vi "Periodic Tasks.vi"(8 "error in":errorcluster) -> ()   [LabVIEW 2019]
doc: "This VI runs in parallel to other tasks. It can contain as many user-defined periodic loops as you need. These can carry out PID or other sorts of timed response."
uses:
  <vilib>/Rock Robotics/WPI/DriverStation/WPI_DriverStationRobotMode2.ctl
  <vilib>/Rock Robotics/WPI/Utilities/WPI_GetSetVariantRefNum.vi
  Robot Global Data.vi
  <vilib>/Rock Robotics/WPI/RobotDrive/WPI_RobotDriveArcadeDrive_Standard(NoSaturation).vi
  <vilib>/Rock Robotics/Network Tables/NT Write Numeric Array.vi
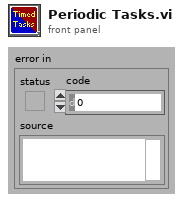
[diagram p1: front panel]
types:
  T1 = typedef "WPI_RobotDriveDevRef.ctl" = cluster{"DevStatus":errorcluster, "Motors[]":T2[], "Square Inputs":bool, "Max Output":dbl}
  T2 = typedef "WPI_MotorControlDeviceRef.ctl" = cluster{"DeviceStatus":errorcluster, "Type":T3, "PWM":cluster{"PWM Channel":T4, "DeadBand":T5}, "CAN":cluster{"Device Number":u8, "SetOutput VI Ref":variant, "GetOutput VI Ref":variant, "Enable VI Ref":variant, "Disable VI Ref":variant, "Data":variant}, "Invert":bool, "DIO PWM":cluster{"PWM \"Enable\" Channel":T4, "DIOChannel":T6, "PWM Rate":dbl}}
  T3 = typedef "WPI_MotorControlType.ctl" = enum16{"PWM", "CAN", "DIO PWM"}
  T4 = typedef "FPGA_DIOPWMChannel.ctl" = enum8{"PWM 0", "PWM 1", "PWM 2", "PWM 3", "PWM 4", "PWM 5", "PWM 6", "PWM 7", "PWM 8", "PWM 9", "PWM MXP 0", "PWM MXP 1", "PWM MXP 2", "PWM MXP 3", "PWM MXP 4", "PWM MXP 5", "PWM MXP 6", "PWM MXP 7", "PWM MXP 8", "PWM MXP 9", "Invalid"}
  T5 = typedef "WPI_PWMDeadband.ctl" = cluster{"Name":string, "maxPositivePwm":i32, "minPositivePwm":i32, "centerPwm":i32, "maxNegativePwm":i32, "minNegativePwm":i32, "angularRange":u16}
  T6 = typedef "FPGA_DIOChannel.ctl" = enum8{"DIO 0", "DIO 1", "DIO 2", "DIO 3", "DIO 4", "DIO 5", "DIO 6", "DIO 7", "DIO 8", "DIO 9", "DIO MXP 0", "DIO MXP 1", "DIO MXP 2", "DIO MXP 3", "DIO MXP 4", "DIO MXP 5", "DIO MXP 6", "DIO MXP 7", "DIO MXP 8", "DIO MXP 9", "DIO MXP 10", "DIO MXP 11", "DIO MXP 12", "DIO MXP 13", "DIO MXP 14", "DIO MXP 15", "SPI Port CS1", "SPI Port CS2", "SPI Port CS3", "SPI Port MISO", "SPI Port MOSI", "Invalid"}
  T7 = typedef "WPI_JoystickDevRef.ctl" = cluster{"Device":T8}
  T8 = typedef "WPI_JoystickDeviceEnum.ctl" = enum16{"USB 0", "USB 1", "USB 2", "USB 3", "USB 4", "USB 5"}
  T9 = cluster{"JoystickDevRef":T7, "RobotDriveDevRef":T1}
  T10 = typedef "WPI_DriverStationRobotMode2.ctl" = enum16{"Autonomous Disabled", "Autonomous Enabled", "Teleop Disabled", "Teleop Enabled", "Disconnected", "Finish", "Test Disabled", "Test Enabled", "Emergency Stopped"}
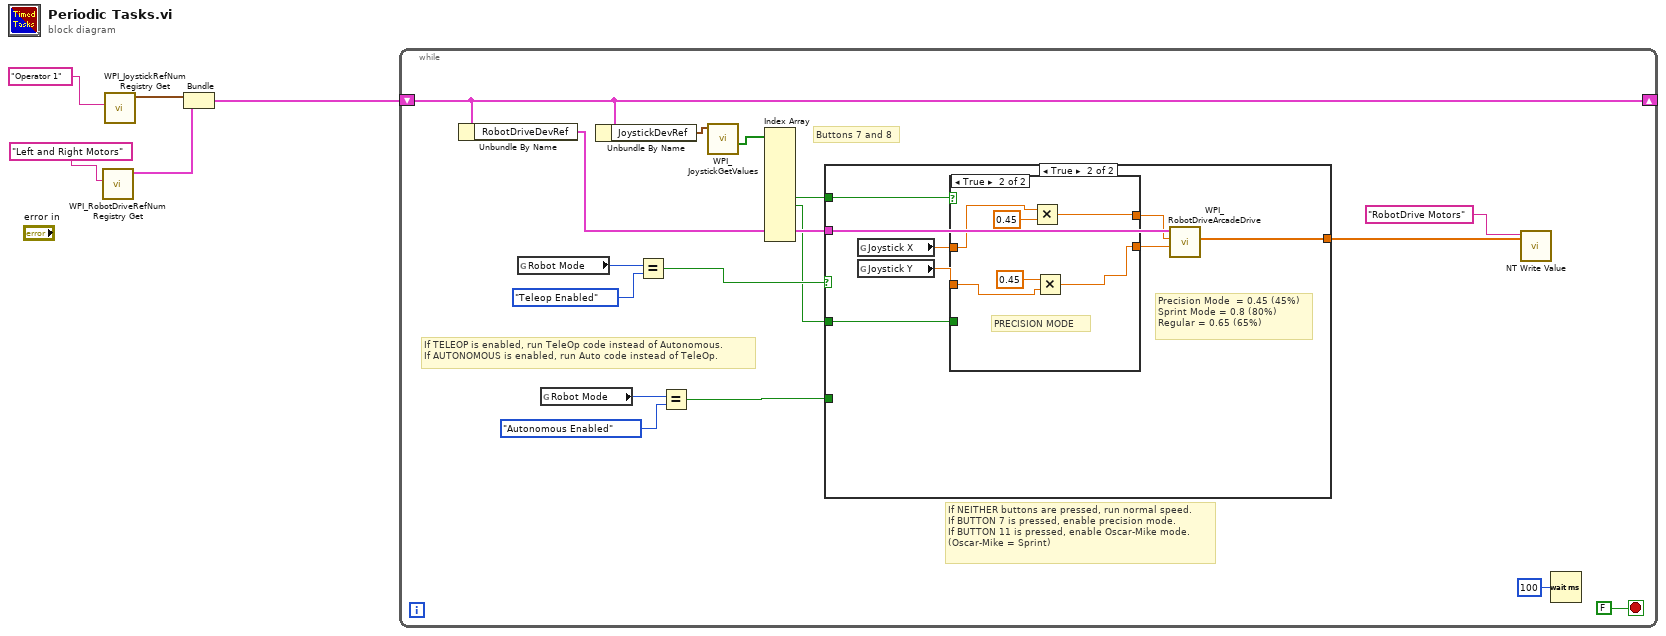
[diagram p0: block diagram]
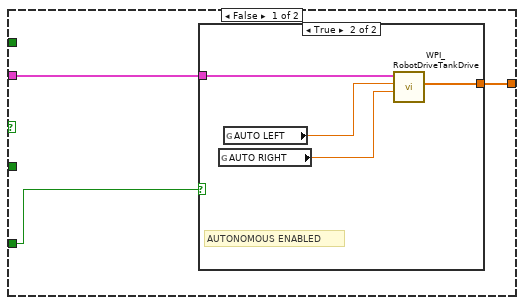
[diagram p2: hidden frame]
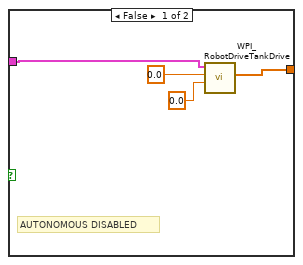
[diagram p3: hidden frame]
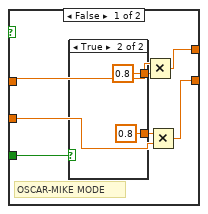
[diagram p4: hidden frame]
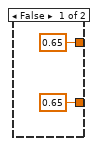
[diagram p5: hidden frame]
diagram:
  n1 = call <vilib>:"WPI_RobotDriveRefNum Registry Get.vi"("refnum name"="Left and Right Motors") -> ("RobotDriveDevRef"=w5:T1)  [unwired: 1 in, 9 out]
  n2 = call <vilib>:"WPI_JoystickRefNum Registry Get.vi"("refnum name"="Operator 1") -> ("JoystickDevRef"=w4:T7)  [unwired: 1 in, 9 out]
  n3 = Bundle("JoystickDevRef"=w4, "RobotDriveDevRef"=w5) -> (w1:T9)  [unwired: 1 out]
  n4 = while {
    shift-right: [w10] -> _
    shift-left: w1 -> [w10]
    stop <- FALSE stop-if-true
    # "If NEITHER buttons are pressed, run normal speed.\nIf BUTTON 7 is pressed, enable precision mode.\nIf BUTTON 11 is pressed, enable Oscar-Mike mode.\n(Oscar-Mike = Sprint)"
    # "Buttons 7 and 8"
    # "If TELEOP is enabled, run TeleOp code instead of Autonomous.\nIf AUTONOMOUS is enabled, run Auto code instead of TeleOp."
    n5 = Unbundle By Name(w10) -> ("RobotDriveDevRef"=w17:T1)
    n6 = global read "Robot Global Data.vi" "Robot Mode"() -> (w15:T10)
    n7 = global read "Robot Global Data.vi" "Robot Mode"() -> (w13:T10)
    n8 = Unbundle By Name(w10) -> ("JoystickDevRef"=w9:T7)
    n9 = Equal?(x=w15, y=WPI_DriverStationRobotMode2."Teleop Enabled") -> (x = y?=w16:bool)
    n10 = Equal?(x=w13, y=WPI_DriverStationRobotMode2."Autonomous Enabled") -> (x = y?=w11:bool)
    n11 = call <vilib>:"WPI_JoystickGetValues.vi"("JoystickDevRef"=w9) -> ("Buttons"=w8:bool[])  [unwired: 6 in, 4 out]
    n12 = Index Array(array=w8) -> (element #7=w7:bool, element #8=w6:bool)  [unwired: 12 in, 10 out]
    n13 = case shown="True" w16 {
      tunnel: [w24 w39] -> w18
      tunnel: w17 -> [w23 w40]
      tunnel: w11 -> [w22 _]
      tunnel: w6 -> [_ w34]
      tunnel: w7 -> [_ w33]
      frame False {
        n14 = case shown="True" w22 {
          tunnel: [w28 w32] -> w24
          tunnel: w23 -> [w25 w30]
          frame False {
            # "AUTONOMOUS DISABLED"
            n15 = call <vilib>:"WPI_RobotDriveTankDrive.vi"("Right axis value"=0.0, "Left axis value"=0.0, "RobotDriveDevRef"=w25) -> ("Motor Values"=w28:dbl[])  [unwired: 6 in, 2 out]
          }
          frame True {
            # "AUTONOMOUS ENABLED"
            n16 = global read "Robot Global Data.vi" "AUTO RIGHT"() -> (w29:dbl)
            n17 = global read "Robot Global Data.vi" "AUTO LEFT"() -> (w31:dbl)
            n18 = call <vilib>:"WPI_RobotDriveTankDrive.vi"("Right axis value"=w29, "Left axis value"=w31, "RobotDriveDevRef"=w30) -> ("Motor Values"=w32:dbl[])  [unwired: 6 in, 2 out]
          }
        }
      }
      frame True {
        # "Precision Mode  = 0.45 (45%)\nSprint Mode = 0.8 (80%)\nRegular = 0.65 (65%)"
        n19 = global read "Robot Global Data.vi" "Joystick X"() -> (w38:dbl)
        n20 = global read "Robot Global Data.vi" "Joystick Y"() -> (w37:dbl)
        n21 = case shown="True" w33 {
          tunnel: w38 -> [w44 w55]
          tunnel: w37 -> [w45 w54]
          tunnel: [w43 w56] -> w36
          tunnel: [w42 w57] -> w35
          tunnel: w34 -> [w41 _]
          frame False {
            # "OSCAR-MIKE MODE"
            n22 = case shown="True" w41 {
              tunnel: [0.65 ("x") 0.8 ("x")] -> w47
              tunnel: [0.65 ("y") 0.8 ("y")] -> w46
              frame False {
              }
              frame True {
              }
            }
            n23 = Multiply(x=w44, y=w46) -> (x*y=w43:dbl)
            n24 = Multiply(x=w47, y=w45) -> (x*y=w42:dbl)
          }
          frame True {
            # "PRECISION MODE"
            n25 = Multiply(x=w55, y=0.45) -> (x*y=w56:dbl)
            n26 = Multiply(x=0.45, y=w54) -> (x*y=w57:dbl)
          }
        }
        n27 = call-poly <vilib>:"WPI_RobotDriveArcadeDrive.vi"("Y axis value"=w35, "X axis value"=w36, "RobotDriveDevRef"=w40) -> ("Motor Values"=w39:dbl[])  [unwired: 6 in, 2 out]
      }
    }
    n28 = call-poly <vilib>:"NT Write Value.vi"("Numeric Array"=w18, "Name"="RobotDrive Motors") -> ()  [unwired: 9 in, 1 out]
    n29 = Wait (ms)(milliseconds to wait=u32 100) -> ()  [unwired: 1 out]
  }
